vi "CMN_KeyVal2Array.vi"(7 "error in (no error)":errorcluster, 8 "separator":string="[,;\\n]", 9 "command in":string) -> (0 "error out":errorcluster, 1 "number of commands":i32, 2 "commands out":string)   [LabVIEW 2016]
doc: "This VI takes an input cmd list separated by commas, and using the \"key=value\" or \"key value\" notation, and return an output multi-line string of type \"key val\". \n\nInput\nvar1=val1, var2=val2 .... varN=valN\n\nOutput\nvar1 val1\nvar2 val2\n...\nvarN valN"
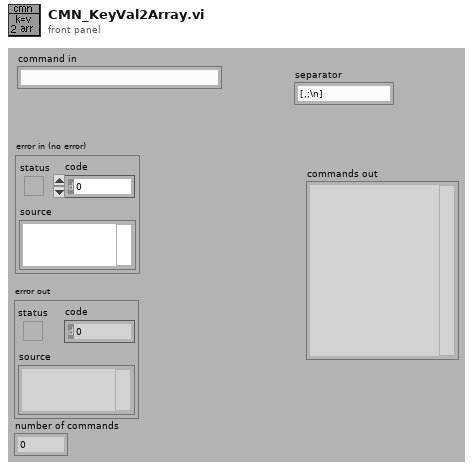
[diagram p1: front panel]
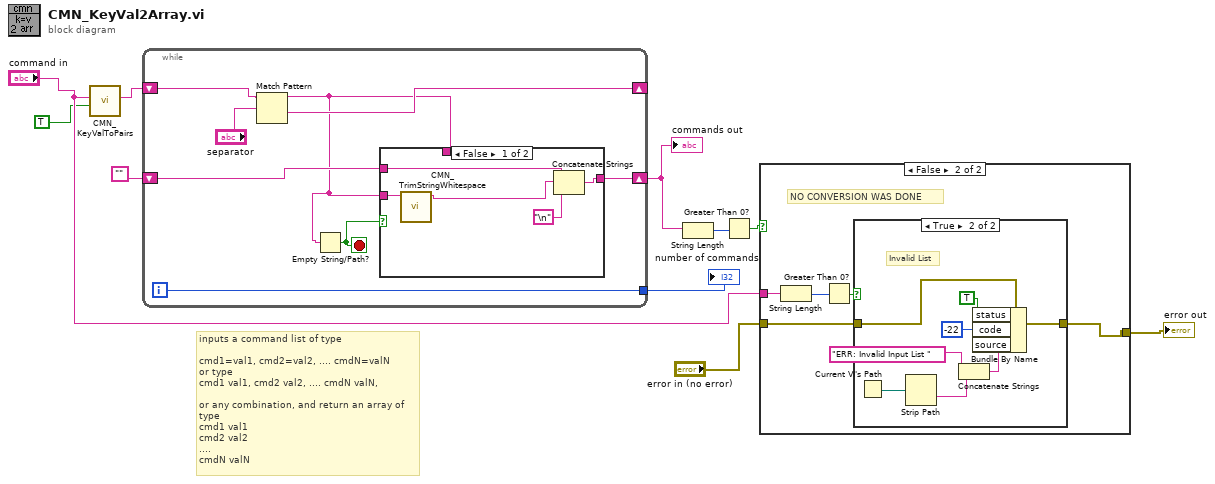
[diagram p0: block diagram]
diagram:
  # "inputs a command list of type\n\ncmd1=val1, cmd2=val2, .... cmdN=valN\nor type\ncmd1 val1, cmd2 val2, .... cmdN valN,\n\nor any combination, and return an array of type\ncmd1 val1\ncmd2 val2\n....\ncmdN valN"
  n1 = call "CMN_KeyValToPairs.vi"("replace all? (F)"=TRUE, "key=value pairs"="command in") -> ("arguments out"=w6:string)  [unwired: 9 out]
  n2 = while {
    shift-right: [w18] -> _
    shift-left: w6 -> [w13]
    shift-right: [w15] -> w3
    shift-left: "" -> [w14]
    tunnel: [w11] -> w1
    i -> [w11]
    stop <- w16 stop-if-true
    n3 = Match Pattern(string=w13, regular expression="separator") -> (before substring=w12:string, after substring=w18:string)  [unwired: 3 out]
    n4 = Empty String/Path?(string/path=w12) -> (empty?=w16:bool)
    n5 = case shown="False" w16 {
      tunnel: w12 -> [w23 _]
      tunnel: w12 -> [_ _]
      tunnel: [w20 w24] -> w15
      tunnel: w14 -> [w22 w24]
      frame False {
        n6 = call "CMN_TrimStringWhitespace.vi"("string"=w23) -> ("trimmed string"=w19:string)  [unwired: 1 in, 8 out]
        n7 = Concatenate Strings(w22, w19, "\n") -> (w20:string)
      }
      frame True {
      }
    }
  }
  "commands out" <- w3
  "number of commands" <- w1
  n8 = String Length(string=w3) -> (length=w2:i32)
  n9 = Greater Than 0?(x=w2) -> (x > 0?=w10:bool)
  n10 = case shown="False" w10 {
    tunnel: "command in" -> [_ w30]
    tunnel: "error in (no error)" -> [w25 w27]
    tunnel: [w25 w26] -> w8
    frame True {
    }
    frame False {
      # "NO CONVERSION WAS DONE"
      n11 = String Length(string=w30) -> (length=w29:i32)
      n12 = Greater Than 0?(x=w29) -> (x > 0?=w28:bool)
      n13 = case shown="True" w28 {
        tunnel: w27 -> [w31 w33]
        tunnel: [w31 w32] -> w26
        frame False {
        }
        frame True {
          # "Invalid List"
          n14 = Current VI's Path() -> (path=w36:path)
          n15 = Strip Path(path=w36) -> (name=w35:string)  [unwired: 1 out]
          n16 = Concatenate Strings("ERR: Invalid Input List " ("string"), w35) -> (w34:string)
          n17 = Bundle By Name(cluster=w33, "status"=TRUE, "code"=-22, "source"=w34) -> (w32:errorcluster)
        }
      }
    }
  }
  "error out" <- w8
